vi "Unknown Connection Error.vi"(8 "error in (no error)":errorcluster, 11 "connection":T1) -> (0 "error out":errorcluster)   [LabVIEW 2017, in "Routing and Faulting Scripting.lvlib"]
uses:
  Routing and Faulting Scripting.lvlib
  Shared/Connection.ctl
  Shared/Routing and Faulting Shared.lvlib
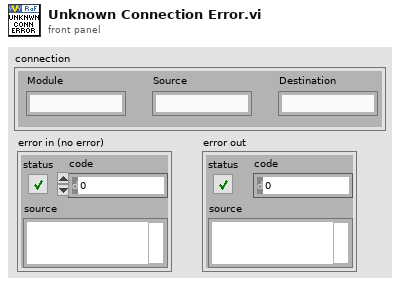
[diagram p1: front panel]
types:
  T1 = typedef "Routing and Faulting Shared.lvlib/Connection.ctl" = cluster{"Module":string, "Source":string, "Destination":string}
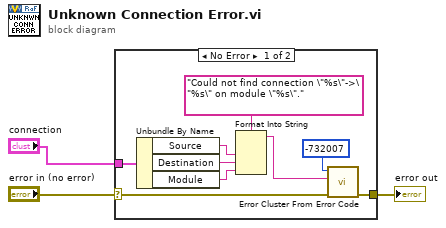
[diagram p0: block diagram]
diagram:
  n1 = case shown="No Error" "error in (no error)" {
    selector: "error in (no error)" -> [w9 w13]
    tunnel: "connection" -> [w7 _]
    tunnel: [w10 w13] -> w2
    frame No Error {
      n2 = Unbundle By Name(w7) -> ("Source"=w6:string, "Destination"=w5:string, "Module"=w4:string)
      n3 = Format Into String(format string="Could not find connection \"%s\"->\"%s\" on module \"%s\".", w6, w5, w4) -> (resulting string=w12:string)  [unwired: 2 in, 1 out]
      n4 = call <vilib>:"Error Cluster From Error Code.vi"("error in (no error)"=w9, "error message (\"\")"=w12, "error code (0)"=-732007) -> ("error out"=w10:errorcluster)  [unwired: 6 in]
    }
    frame Error {
    }
  }
  "error out" <- w2
